vi "Configure Input Parameters.vi"(0 "VISA resource name":refnum<visa-resource-name>, 1 "Input Name (\"\")":string, 2 "Enable \nCompensation (F: Off)":bool, 5 "Input (0:A)":u16(ring) items=["A", "B"], 7 "Sensor Type and Range (0:Disabled)":u16(ring) items=["Disabled", "Diode 2.5 V (Silicon)", "Diode 10 V (GaAlAs)", "PTC RTD Autorange", "PTC RTD 10 Ohm", "PTC RTD 30 Ohm", "PTC RTD 100 Ohm", "PTC RTD 300 Ohm", "PTC RTD 1 kOhm", "PTC RTD 3 kOhm", "PTC RTD 10 kOhm", "NTC RTD Autorange", "NTC RTD 10 Ohm", "NTC RTD 30 Ohm", "NTC RTD 100 Ohm", "NTC RTD 300 Ohm", "NTC RTD 1 kOhm", "NTC RTD 3 kOhm", "NTC RTD 10 kOhm", "NTC RTD 30 kOhm", "NTC RTD 100 kOhm", "Thermocouple"], 9 "Diode Current (0:10 uA)":u16(ring) items=["10 uA", "1 mA"], 11 "error in (no error)":errorcluster, 12 "Preferred Units (1:Kelvin)":u16(ring)=1 items=["Kelvin"=1, "Celsius"=2, "Sensor Units"=3], 13 "Curve (0:None)":u16(ring) items=["None"=0, "DT-470"=1, "DT-670"=2, "DT-500-D"=3, "DT-500-E1"=4, "PT-100"=6, "PT-1000"=7, "RX-102A-AA"=8, "RX-202A-AA"=9, "Type K"=12, "Type E"=13, "Type T"=14, "AuFe 0.03%"=15, "AuFe 0.07%"=16, "User 21"=21, "User 22"=22, "User 23"=23, "User 24"=24, "User 25"=25, "User 26"=26, "User 27"=27, "User 28"=28, "User 29"=29, "User 30"=30, "User 31"=31, "User 32"=32, "User 33"=33, "User 34"=34, "User 35"=35, "User 36"=36, "User 37"=37, "User 38"=38, "User 39"=39, "User 40"=40, "User 41"=41, "User 42"=42, "User 43"=43, "User 44"=44, "User 45"=45, "User 46"=46, "User 47"=47, "User 48"=48, "User 49"=49, "User 50"=50, "User 51"=51, "User 52"=52, "User 53"=53, "User 54"=54, "User 55"=55, "User 56"=56, "User 57"=57, "User 58"=58, "User 59"=59], 14 "Temperature Limit (0)":u16) -> (4 "VISA resource name out":refnum<visa-resource-name>, 15 "error out":errorcluster)   [LabVIEW 2015, in "Lake Shore 335.lvlib"]
doc: "Configures the sensor input parameters. The Model 335 supports a variety of temperature sensors sold by Lake Shore and other manufacturers. An appropriate sensor type must be selected for each of the four inputs. If the exact sensor model is not shown, use the sensor input types chart in section 4 of the 335 User's Manual."
uses:
  <instrlib>/Lake Shore 335/Lake Shore 335.lvlib
  Instance           1 34Saved   Configure Input Parameters .vi
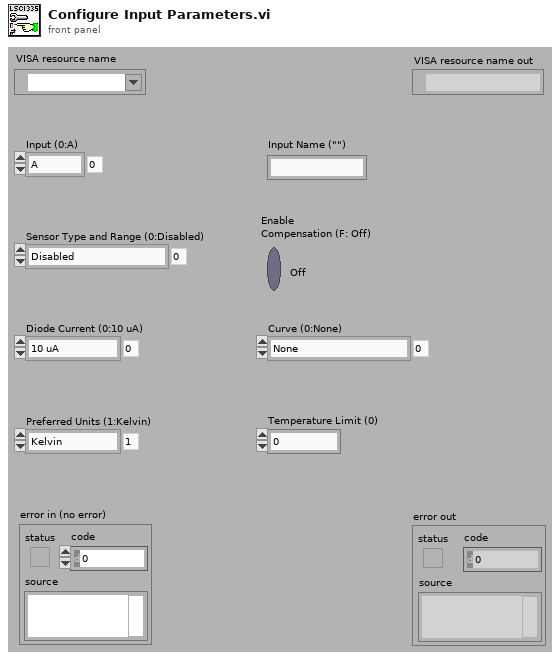
[diagram p1: front panel]
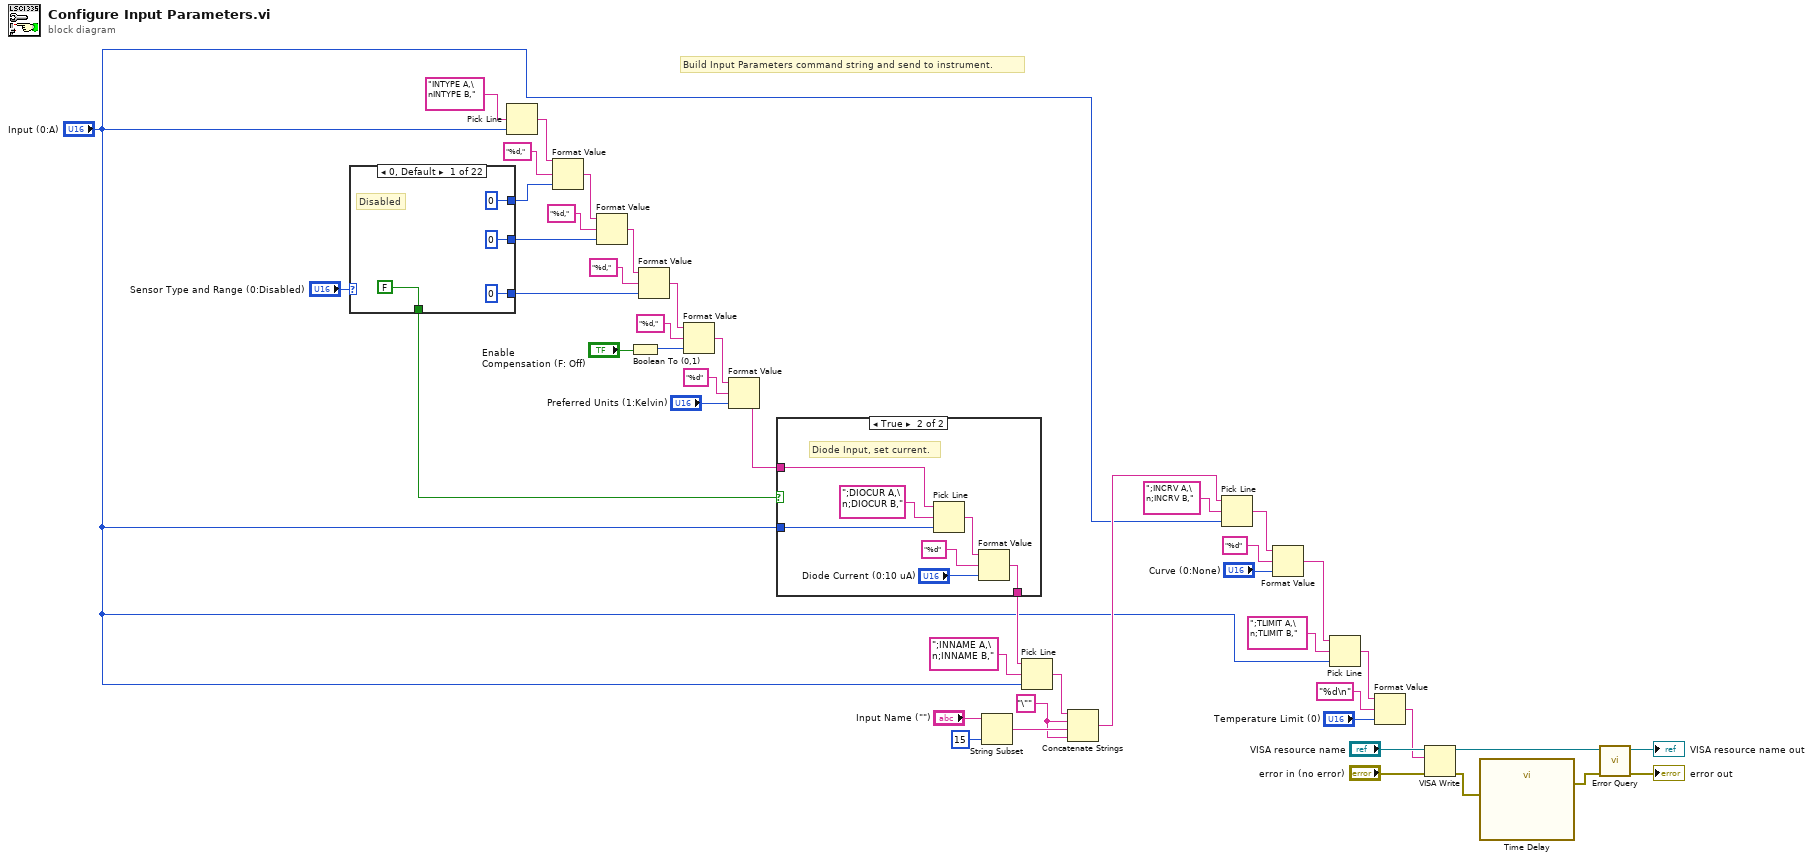
[diagram p0: block diagram]
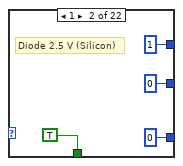
[diagram p3: hidden frame]
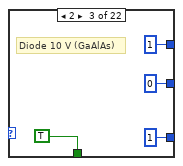
[diagram p4: hidden frame]
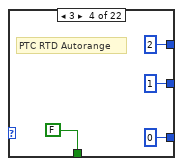
[diagram p5: hidden frame]
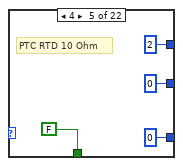
[diagram p6: hidden frame]
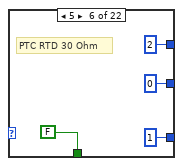
[diagram p7: hidden frame]
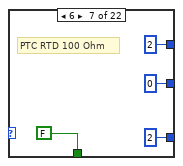
[diagram p8: hidden frame]
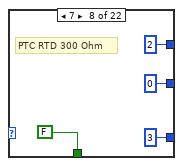
[diagram p9: hidden frame]
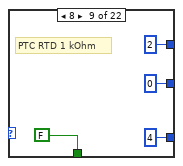
[diagram p10: hidden frame]
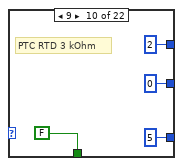
[diagram p11: hidden frame]
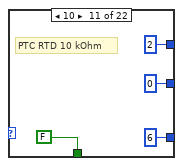
[diagram p12: hidden frame]
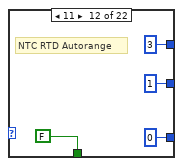
[diagram p13: hidden frame]
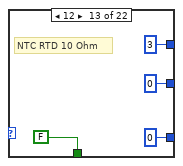
[diagram p14: hidden frame]
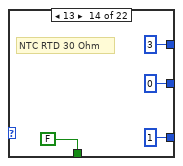
[diagram p15: hidden frame]
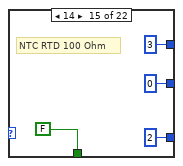
[diagram p16: hidden frame]
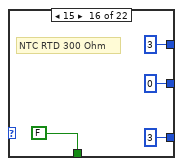
[diagram p17: hidden frame]
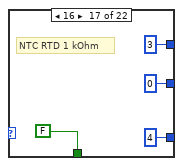
[diagram p18: hidden frame]
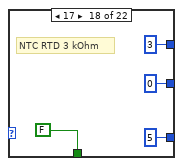
[diagram p19: hidden frame]
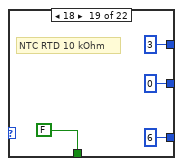
[diagram p20: hidden frame]
diagram:
  w9 = "\""
  # "Build Input Parameters command string and send to instrument."
  n1 = case shown="0, Default" "Sensor Type and Range (0:Disabled)" {
    tunnel: [0 1 1 2 2 2 2 2 2 2 2 3 3 3 3 3 3 3 3 3 3 4] -> w20
    tunnel: [0 0 0 1 0 0 0 0 0 0 0 1 0 0 0 0 0 0 0 0 0 0] -> w19
    tunnel: [0 0 1 0 0 1 2 3 4 5 6 0 0 1 2 3 4 5 6 7 8 0] -> w18
    tunnel: [FALSE TRUE TRUE FALSE FALSE FALSE FALSE FALSE FALSE FALSE FALSE FALSE FALSE FALSE FALSE FALSE FALSE FALSE FALSE FALSE FALSE FALSE] -> w2
    frame 0, Default {
      # "Disabled"
    }
    frame 1 {
      # "Diode 2.5 V (Silicon)"
    }
    frame 2 {
      # "Diode 10 V (GaAlAs)"
    }
    frame 3 {
      # "PTC RTD Autorange"
    }
    frame 4 {
      # "PTC RTD 10 Ohm"
    }
    frame 5 {
      # "PTC RTD 30 Ohm"
    }
    frame 6 {
      # "PTC RTD 100 Ohm"
    }
    frame 7 {
      # "PTC RTD 300 Ohm"
    }
    frame 8 {
      # "PTC RTD 1 kOhm"
    }
    frame 9 {
      # "PTC RTD 3 kOhm"
    }
    frame 10 {
      # "PTC RTD 10 kOhm"
    }
    frame 11 {
      # "NTC RTD Autorange"
    }
    frame 12 {
      # "NTC RTD 10 Ohm"
    }
    frame 13 {
      # "NTC RTD 30 Ohm"
    }
    frame 14 {
      # "NTC RTD 100 Ohm"
    }
    frame 15 {
      # "NTC RTD 300 Ohm"
    }
    frame 16 {
      # "NTC RTD 1 kOhm"
    }
    frame 17 {
      # "NTC RTD 3 kOhm"
    }
    frame 18 {
      # "NTC RTD 10 kOhm"
    }
    frame 19 {
      # "NTC RTD 30 kOhm"
    }
    frame 20 {
      # "NTC RTD 100 kOhm"
    }
    frame 21 {
      # "Thermocouple"
    }
  }
  n2 = Pick Line(multi-line string="INTYPE A,\nINTYPE B,", line index="Input (0:A)") -> (output string=w38:string)  [unwired: 1 in]
  n3 = Format Value(string ("")=w38, format string="%d,", value (0)=w20) -> (output string=w28:string)
  n4 = Format Value(string ("")=w28, format string="%d,", value (0)=w19) -> (output string=w26:string)
  n5 = Boolean To (0,1)(Boolean="Enable \nCompensation (F: Off)") -> (0, 1=w35:i16)
  n6 = Format Value(string ("")=w26, format string="%d,", value (0)=w18) -> (output string=w25:string)
  n7 = Format Value(string ("")=w25, format string="%d,", value (0)=w35) -> (output string=w23:string)
  n8 = Format Value(string ("")=w23, format string="%d", value (0)="Preferred Units (1:Kelvin)") -> (output string=w3:string)
  n9 = case shown="True" w2 {
    tunnel: [w135 w142] -> w4
    tunnel: w3 -> [w135 w137]
    tunnel: "Input (0:A)" -> [_ w136]
    frame False {
      # "Not Diode Input, do not set current."
    }
    frame True {
      # "Diode Input, set current."
      n10 = Pick Line(string ("")=w137, multi-line string=";DIOCUR A,\n;DIOCUR B,", line index=w136) -> (output string=w140:string)
      n11 = Format Value(string ("")=w140, format string="%d", value (0)="Diode Current (0:10 uA)") -> (output string=w142:string)
    }
  }
  n12 = String Subset(string="Input Name (\"\")", length (rest)=15) -> (substring=w10:string)  [unwired: 1 in]
  n13 = Pick Line(string ("")=w4, multi-line string=";INNAME A,\n;INNAME B,", line index="Input (0:A)") -> (output string=w15:string)
  n14 = Concatenate Strings(w15, w9, w10, w9) -> (w5:string)
  n15 = Pick Line(string ("")=w5, multi-line string=";INCRV A,\n;INCRV B,", line index="Input (0:A)") -> (output string=w33:string)
  n16 = Format Value(string ("")=w33, format string="%d", value (0)="Curve (0:None)") -> (output string=w6:string)
  n17 = Pick Line(string ("")=w6, multi-line string=";TLIMIT A,\n;TLIMIT B,", line index="Input (0:A)") -> (output string=w12:string)
  n18 = Format Value(string ("")=w12, format string="%d\n", value (0)="Temperature Limit (0)") -> (output string=w7:string)
  n19 = VISA Write(VISA resource name="VISA resource name", write buffer=w7, error in (no error)="error in (no error)") -> (VISA resource name out=w44:refnum<visa-resource-name>, error out=w31:errorcluster)  [unwired: 1 out]
  n20 = call "Time Delay"("error in (no error)"=w31) -> ("error out"=w30:errorcluster)  [unwired: 10 in]
  n21 = call <instrlib>:"Error Query.vi"("error in (no error)"=w30, "VISA resource name"=w44) -> ("error out"=→"error out":errorcluster, "VISA resource name out"=→"VISA resource name out":refnum<visa-resource-name>)  [unwired: 7 in, 1 out]
